vi "startVideo.vi"(8 "error in (no error)":errorcluster, 11 "AtomChipHWC in":refnum<class "AtomChipHWC.lvclass">) -> (0 "error out":errorcluster, 3 "AtomChipHWC out":refnum<class "AtomChipHWC.lvclass">)   [LabVIEW 2009, in "Hardware.lvlib" / "HWControllers.lvlib" / "AtomChipHWC.lvclass"]
uses:
  AtomChipHWC.lvclass
  HardwareConfiguration/HWConfiguration.lvclass
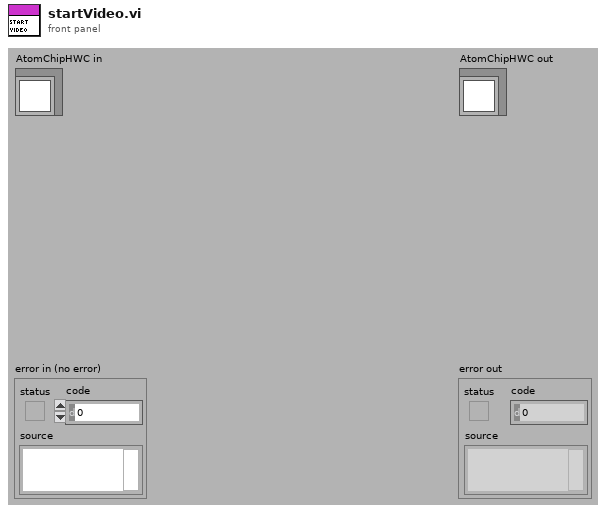
[diagram p1: front panel]
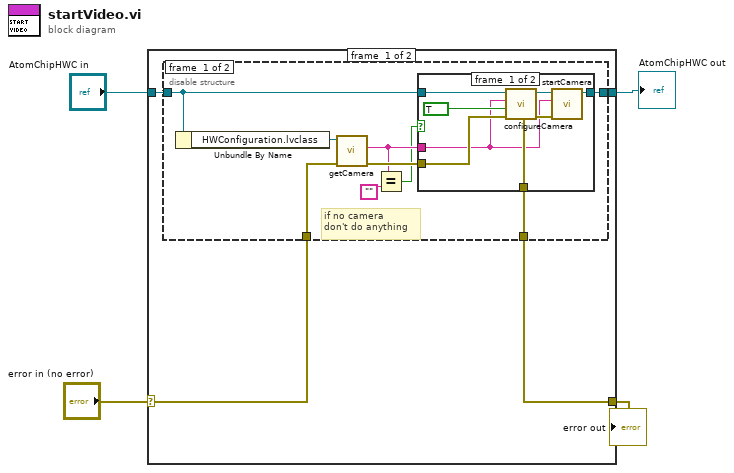
[diagram p0: block diagram]
diagram:
  n1 = case shown="No Error" "error in (no error)" {
    selector: "error in (no error)" -> [w8 w30]
    tunnel: [w6 w31] -> w3
    tunnel: "AtomChipHWC in" -> [w7 w31]
    tunnel: [w5 w30] -> w1
    frame #0 {
      n2 = disable-structure shown="Enabled" {
        disable-tunnel: w8 -> [w16 w29]
        disable-tunnel: w7 -> [w15 w28]
        disable-tunnel: [w13 w28] -> w6
        disable-tunnel: [w12 w29] -> w5
        frame #0 {
          # "if no camera\ndon't do anything"
          n3 = Unbundle By Name(w15) -> ("HWConfiguration.lvclass"=w17:refnum<class "HWConfiguration.lvclass">)
          n4 = call-dynamic "getCamera.vi"("error in (no error)"=w16, "HWConfiguration.lvclass in"=w17) -> ("error out"=w14:errorcluster, "camera"=w11:string)  [unwired: 7 in, 1 out]
          n5 = Equal?(x=w11, y="") -> (x = y?=w9:bool)
          n6 = case shown="False" w9 {
            tunnel: w15 -> [w25 w27]
            tunnel: w14 -> [w24 w26]
            tunnel: [w21 w27] -> w13
            tunnel: [w20 w26] -> w12
            tunnel: w11 -> [w18 _]
            frame #0 {
              n7 = call "configureCamera.vi"("error in (no error)"=w24, "video"=TRUE, "device"=w18, "AtomChipHWC in"=w25) -> ("error out"=w23:errorcluster, "AtomChipHWC out"=w22:refnum<class "AtomChipHWC.lvclass">)  [unwired: 6 in]
              n8 = call "startCamera.vi"("error in (no error)"=w23, "camera"=w18, "AtomChipHWC in"=w22) -> ("error out"=w20:errorcluster, "AtomChipHWC out"=w21:refnum<class "AtomChipHWC.lvclass">)  [unwired: 7 in]
            }
            frame #1 {
            }
          }
        }
        frame #1 {
        }
      }
    }
    frame #1 {
    }
  }
  "error out" <- w1
  "AtomChipHWC out" <- w3
